vi "Curtin_SaveColor.vi"(9 "Color Name":string) -> (1 "New Color":string, 2 "Good?":bool)   [LabVIEW 2022 SP3]
panel:
  in  "Cancel Button":bool
  in  "OK Button":bool
  # "Enter Color Name"
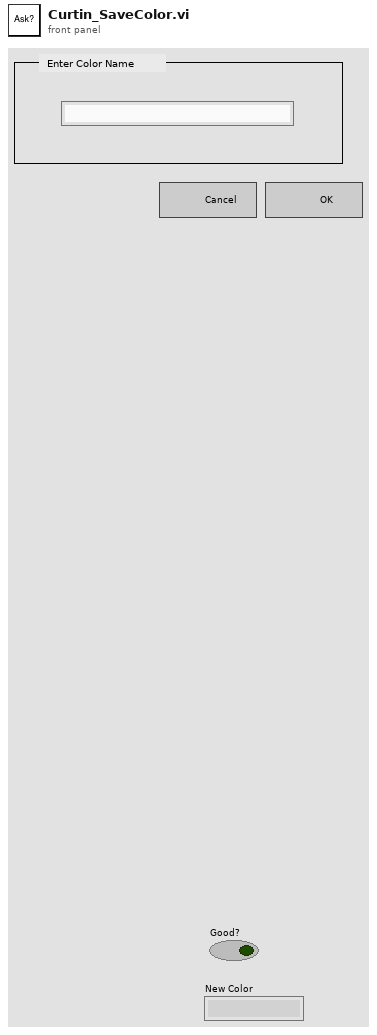
[diagram p1: front panel]
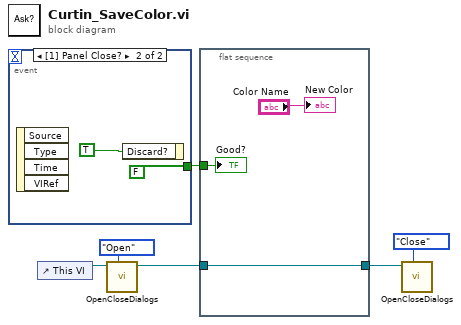
[diagram p0: block diagram]
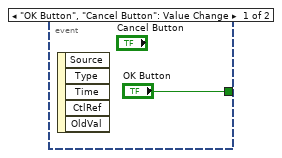
[diagram p2: hidden frame]
diagram:
  n1 = event shown="[1] Panel Close?" {
    selector: _ -> [_ _]
    dyn-events: _ -> [_ _]
    timeout: _ -> [_ _]
    tunnel: ["OK Button" FALSE ("Discard?")] -> w6
    event "OK Button", "Cancel Button": Value Change {
      n2 = event-data() -> ()  [unwired: 1 in, 5 out]
    }
    event Panel Close? {
      n3 = event-data() -> ()  [unwired: 1 in, 4 out]
      n4 = event-data("Discard?"=TRUE) -> ()  [unwired: 1 in, 1 out]
    }
  }
  n5 = control-ref of="This VI"() -> (w4:refnum<vi>)
  n6 = call "OpenCloseDialogs.vi"("Task"=enum16{"Open", "Close"}."Open", "VI in"=w4) -> ("VI out"=w1:refnum<vi>)  [unwired: 8 in, 1 out]
  n7 = flat-sequence {
    tunnel: w6 -> [w12]
    tunnel: [w10] -> w2
    tunnel: w1 -> [w10]
    frame #0 {
      "Good?" <- w12
      "New Color" <- "Color Name"
    }
  }
  n8 = call "OpenCloseDialogs.vi"("Task"=enum16{"Open", "Close"}."Close", "VI in"=w2) -> ()  [unwired: 8 in, 2 out]
